vi "Magazine_Set.vi"   [LabVIEW 2020]
uses:
  Magazine_Control_States.ctl
  Globals/Magazine_Globals.vi
types:
  T1 = typedef "Magazine_Control_States.ctl" = enum16{"No-Op", "Manual_Control", "Load", "Firing"}
  T2 = typedef "Magazine_Cluster.ctl" = cluster{"Control_States":T1, "Manual_Magazine":dbl, "Auto_Magazine":bool}
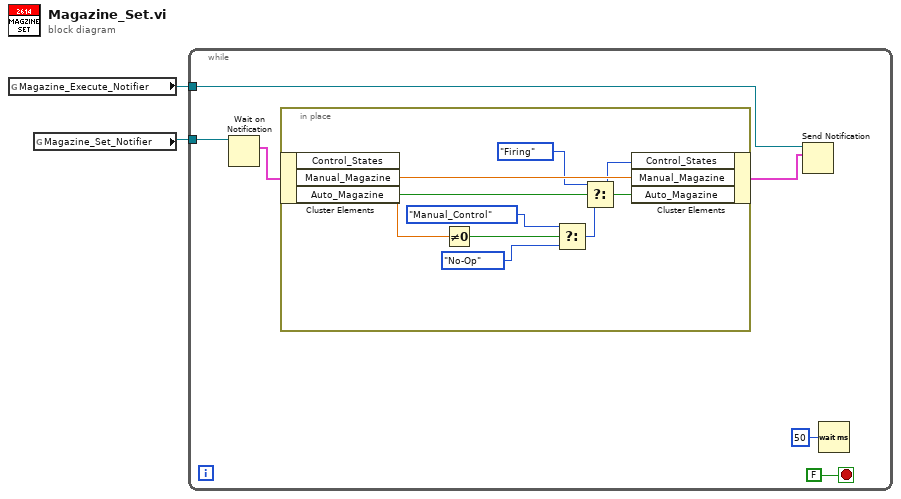
[diagram p0: block diagram]
diagram:
  n1 = global read "Magazine_Globals.vi" "Magazine_Execute_Notifier"() -> (w2:refnum<notifier>)
  n2 = global read "Magazine_Globals.vi" "Magazine_Set_Notifier"() -> (w1:refnum<notifier>)
  n3 = while {
    tunnel: w1 -> [w8]
    tunnel: w2 -> [w4]
    stop <- FALSE stop-if-true
    n4 = Wait on Notification(notifier=w8) -> (notification=w5:T2)  [unwired: 3 in, 3 out]
    n5 = in-place {
      n6 = in-place-cluster #1(w5) -> ("Manual_Magazine"=w13:dbl, "Auto_Magazine"=w9:bool)  [unwired: 1 out]
      n7 = Not Equal To 0?(x=w13) -> (x != 0?=w14:bool)
      n8 = Select(t=Magazine_Control_States."Manual_Control" ("Control_States"), s=w14, f=Magazine_Control_States."No-Op" ("Control_States")) -> (s? t:f=w12:T1)
      n9 = Select(t=Magazine_Control_States."Firing" ("Control_States"), s=w9, f=w12) -> (s? t:f=w10:T1)
      n10 = in-place-cluster #1("Control_States"=w10, "Manual_Magazine"=w13, "Auto_Magazine"=w9) -> (w3:T2)
    }
    n11 = Send Notification(notification=w3, notifier=w4) -> ()  [unwired: 1 in, 2 out]
    n12 = Wait (ms)(milliseconds to wait=u32 50) -> ()  [unwired: 1 out]
  }
